vi "start_pulses.vi"() -> ()   [LabVIEW 2012]
panel:
  in  "stop":bool
  out "Current Amplitude":dbl=0.031
  in  "Amplitude Step (mV)":dbl=2.0
  in  "Start amplitude (mV)":dbl=4.0
  in  "Stop Freq (kHz)":dbl=300.0
  in  "Start Freq (kHz)":dbl=175.0
  in  "Length of pulse (s)":dbl=1.0
  in  "Time betweeen (s)":dbl
  in  "Number of pulses":u16=1
  # "VI to pulse HP3325a generator (for use with piezo launcher)"
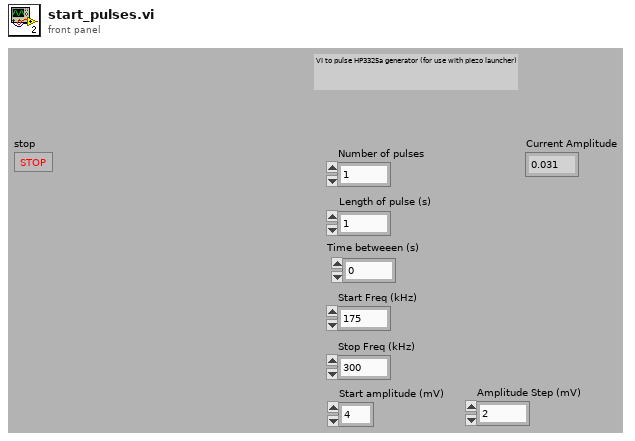
[diagram p1: front panel]
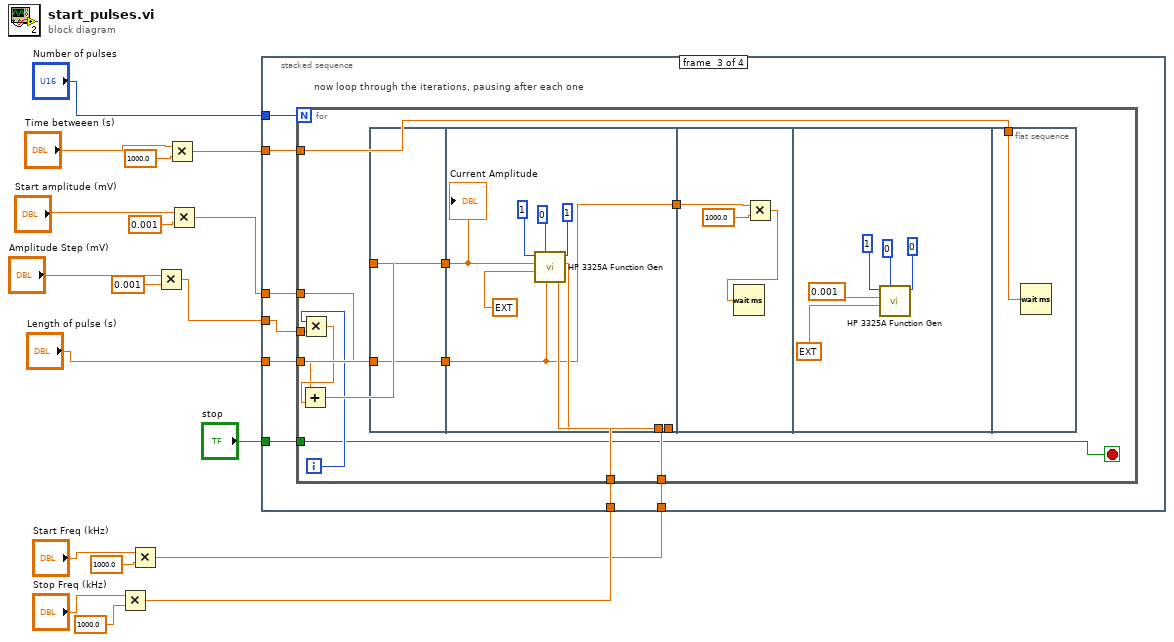
[diagram p0: block diagram]
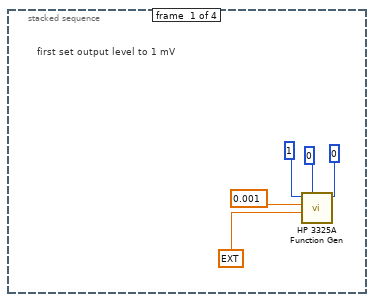
[diagram p2: hidden frame]
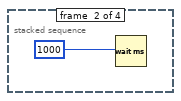
[diagram p3: hidden frame]
diagram:
  n1 = Multiply(x="Stop Freq (kHz)", y=1000.0) -> (x*y=w12:dbl)
  n2 = Multiply(x="Start Freq (kHz)", y=1000.0) -> (x*y=w11:dbl)
  n3 = Multiply(x="Amplitude Step (mV)", y=0.001) -> (x*y=w2:dbl)
  n4 = Multiply(x="Time betweeen (s)", y=1000.0) -> (x*y=w5:dbl)
  n5 = Multiply(x="Start amplitude (mV)", y=0.001) -> (x*y=w8:dbl)
  n6 = stacked-sequence {
    tunnel: "Number of pulses" -> [_ _ w32 _]
    tunnel: w8 -> [_ _ w31 _]
    tunnel: "Length of pulse (s)" -> [_ _ w30 _]
    tunnel: w12 -> [_ _ w29 _]
    tunnel: w11 -> [_ _ w28 _]
    tunnel: w5 -> [_ _ w27 _]
    tunnel: w2 -> [_ _ w26 _]
    tunnel: "stop" -> [_ _ w25 _]
    frame #0 {
      # "first set output level to 1 mV"
      n7 = call "HP 3325A Function Gen.vi"("sweep function (none:0)"=0, "modulation (off:0)"=0, "offset (V)"=ext 0.0, "amplitude (V)"=0.001, "signal type (dc:0)"=i16 1) -> ()  [unwired: 5 in]
    }
    frame #1 {
      n8 = Wait (ms)(milliseconds to wait=1000) -> ()  [unwired: 1 out]
    }
    frame #2 {
      # "now loop through the iterations, pausing after each one"
      n9 = for {
        N: w32 -> [_]
        tunnel: w31 -> [w38]
        tunnel: w30 -> [w40]
        tunnel: w29 -> [w45]
        tunnel: w28 -> [w44]
        tunnel: w27 -> [w43]
        tunnel: w26 -> [w41]
        tunnel: w25 -> [w33]
        i -> [w36]
        stop <- w33 stop-if-true
        n10 = Multiply(x=w36, y=w41) -> (x*y=w39:dbl)
        n11 = Add(x=w38, y=w39) -> (x+y=w37:dbl)
        n12 = flat-sequence {
          tunnel: w37 -> [w46]
          tunnel: w40 -> [w47]
          tunnel: [w47] -> w35
          tunnel: [w46] -> w34
          tunnel: w45 -> [w52]
          tunnel: w44 -> [w51]
          tunnel: [w49] -> w42
          tunnel: w35 -> [w49]
          tunnel: w34 -> [w48]
          tunnel: w42 -> [w57]
          tunnel: w43 -> [w64]
          frame #0 {
          }
          frame #1 {
            n13 = call "HP 3325A Function Gen.vi"("stop"=w52, "start"=w51, "sweep function (none:0)"=1, "sweep time (S)"=w49, "modulation (off:0)"=0, "offset (V)"=ext 0.0, "amplitude (V)"=w48, "signal type (dc:0)"=i16 1) -> ()  [unwired: 2 in]
            "Current Amplitude" <- w48
          }
          frame #2 {
            n14 = Multiply(x=w57, y=1000.0) -> (x*y=w56:dbl)
            n15 = Wait (ms)(milliseconds to wait=w56) -> ()  [unwired: 1 out]
          }
          frame #3 {
            n16 = call "HP 3325A Function Gen.vi"("sweep function (none:0)"=0, "modulation (off:0)"=0, "offset (V)"=ext 0.0, "amplitude (V)"=0.001, "signal type (dc:0)"=i16 1) -> ()  [unwired: 5 in]
          }
          frame #4 {
            n17 = Wait (ms)(milliseconds to wait=w64) -> ()  [unwired: 1 out]
          }
        }
      }
    }
    frame #3 {
    }
  }
